vi "Calculator.vi"() -> ()   [LabVIEW 2018]
panel:
  out "Numeric 3":dbl
  in  "Function":dbl(slide) scale=0.0..3.0
  in  "Numeric 2":dbl
  in  "Numeric":dbl
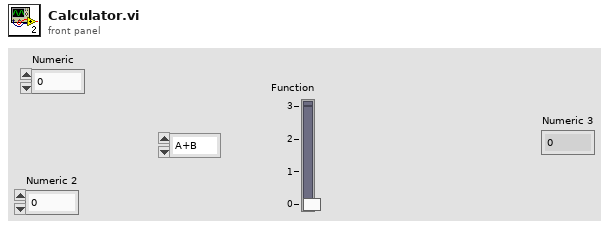
[diagram p1: front panel]
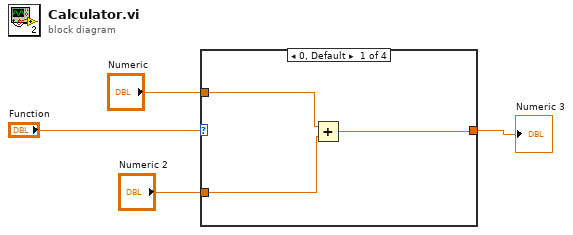
[diagram p0: block diagram]
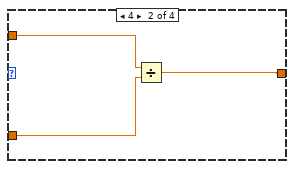
[diagram p2: hidden frame]
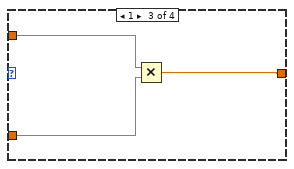
[diagram p3: hidden frame]
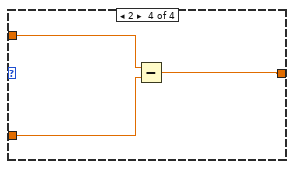
[diagram p4: hidden frame]
diagram:
  n1 = case shown="0, Default" "Function" {
    tunnel: "Numeric" -> [w6 w9 w12 w15]
    tunnel: "Numeric 2" -> [w5 w8 w11 w14]
    tunnel: [w7 w10 w13 w16] -> w1
    frame 0, Default {
      n2 = Add(x=w6, y=w5) -> (x+y=w7:dbl)
    }
    frame 4 {
      n3 = Divide(x=w9, y=w8) -> (x/y=w10:dbl)
    }
    frame 1 {
      n4 = Multiply(x=w12, y=w11) -> (x*y=w13:dbl)
    }
    frame 2 {
      n5 = Subtract(x=w15, y=w14) -> (x-y=w16:dbl)
    }
  }
  "Numeric 3" <- w1
